vi "获取CPUID.vi"(8 "error in (no error)":errorcluster caption="错误输入（无错误）") -> (0 "error out":errorcluster caption="错误输出", 3 "CPU ID":string)   [LabVIEW 2013]
panel:
  out "standard output":string caption="标准输出"
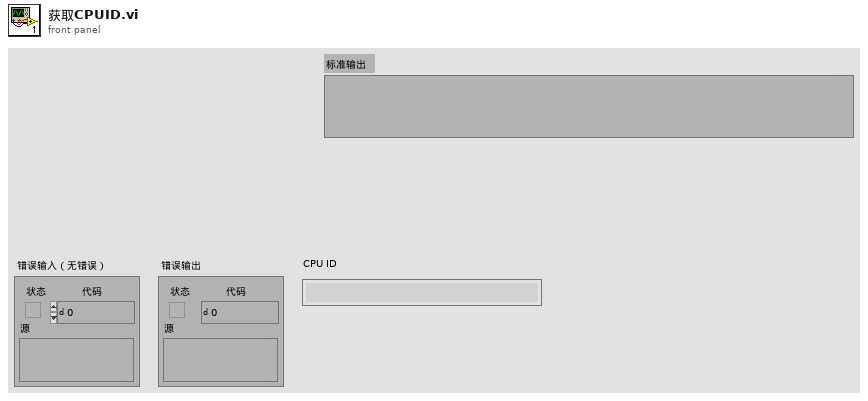
[diagram p1: front panel]
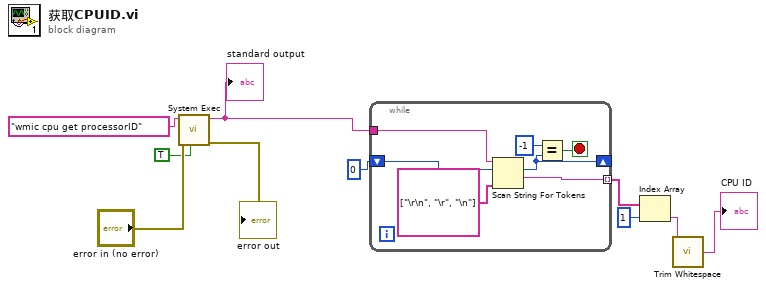
[diagram p0: block diagram]
diagram:
  n1 = call <vilib>:"System Exec.vi"("run minimized? (F)"=TRUE, "error in (no error)"="error in (no error)", "command line"="wmic cpu get processorID" ("standard input")) -> ("error out"=→"error out":errorcluster, "standard output"=w6:string)  [unwired: 5 in, 2 out]
  "standard output" <- w6
  n2 = while {
    tunnel: w6 -> [w17]
    shift-right: [w12] -> _
    shift-left: 0 ("offset past token") -> [w15]
    tunnel: [w13] -> w5 mode=indexing
    stop <- w14 stop-if-true
    n3 = Scan String For Tokens(6:string[] ["\r\n", "\r", "\n"] ("delimiters (\\s,\\t,\\r,\\n)"), 8:w15, 9:w17) -> (1:w13:string, 2:w12:i32)  [unwired: 3 in, 2 out]
    n4 = Equal?(x=-1 ("y"), y=w12) -> (x = y?=w14:bool)
  }
  n5 = Index Array(array=w5, index=1 ("索引")) -> (element=w2:string)
  n6 = call <vilib>:"Trim Whitespace.vi"("string"=w2) -> ("trimmed string"=→"CPU ID":string)  [unwired: 1 in]
